vi "gentec-M-Link.Delay.vi"(0 "VISA resource In":refnum<visa-resource-name>, 2 "delay (100ms)":u32=100, 5 "error in (no error)":errorcluster) -> (14 "VISA resource Out":refnum<visa-resource-name>, 19 "error out":errorcluster)   [LabVIEW 2014, in "gentec-M-Link - Driver.lvlib"]
doc: "This VI sets a delay (in ms)."
uses:
  gentec-M-Link - Driver.lvlib
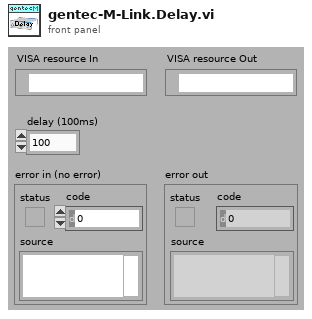
[diagram p1: front panel]
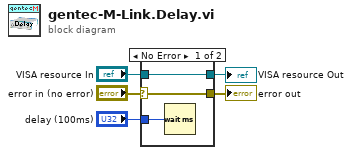
[diagram p0: block diagram]
diagram:
  n1 = case shown="No Error" "error in (no error)" {
    selector: "error in (no error)" -> [w8 w10]
    tunnel: [w8 w10] -> w4
    tunnel: "VISA resource In" -> [w7 w9]
    tunnel: [w7 w9] -> w2
    tunnel: "delay (100ms)" -> [w6 _]
    frame No Error {
      n2 = Wait (ms)(milliseconds to wait=w6) -> ()  [unwired: 1 out]
    }
    frame Error {
    }
  }
  "error out" <- w4
  "VISA resource Out" <- w2
